vi "Read Measurement.vi"   [LabVIEW 2017, in "Keithley 2600 Series.lvlib"]
doc: "Returns one or more measurements."
uses:
  <instrlib>/Keithley 2600 Series/Keithley 2600 Series.lvlib
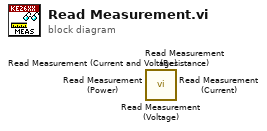
[diagram p0: block diagram]
diagram:
  n1 = call <instrlib>:"Read Measurement (Voltage).vi"() -> ()  [unwired: 8 in, 4 out]
  n2 = call <instrlib>:"Read Measurement (Resistance).vi"() -> ()  [unwired: 8 in, 4 out]
  n3 = call <instrlib>:"Read Measurement (Power).vi"() -> ()  [unwired: 8 in, 4 out]
  n4 = call <instrlib>:"Read Measurement (Current).vi"() -> ()  [unwired: 8 in, 4 out]
  n5 = call <instrlib>:"Read Measurement (Current and Voltage).vi"() -> ()  [unwired: 6 in, 6 out]
